vi "send_trigger.vi"(8 "error in (no error)":errorcluster, 11 "GenericStimulator in":refnum<class "GenericStimulator.lvclass">) -> (0 "error out":errorcluster, 3 "GenericStimulator out":refnum<class "GenericStimulator.lvclass">)   [LabVIEW 2010, in "GenericStimulator.lvclass"]
uses:
  GenericStimulator.lvclass
  trigger_enum.ctl
  common/classes/GenericToplevelComponent/GenericToplevelComponent/trigger_type_enum.ctl
panel:
  in  "trigger":T1
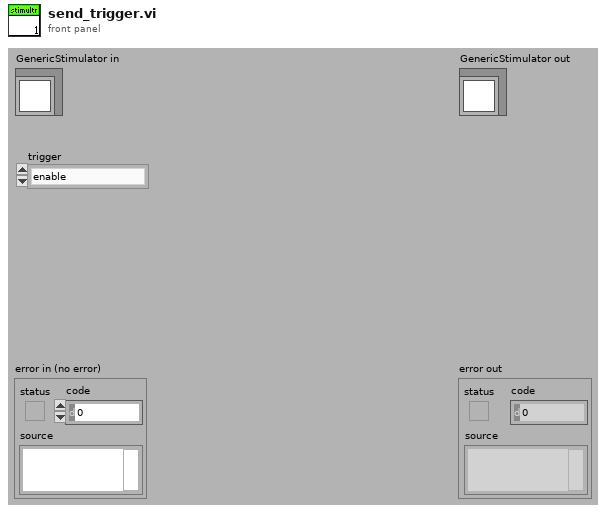
[diagram p1: front panel]
types:
  T1 = typedef "GenericStimulator.lvclass/trigger_enum.ctl" = enum16{"enable", "disable"}
  T2 = typedef "trigger_type_enum.ctl" = enum8{"external", "internal", "common"}
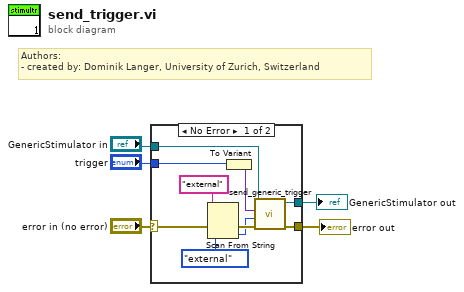
[diagram p0: block diagram]
diagram:
  # "Authors: \n- created by: Dominik Langer, University of Zurich, Switzerland"
  n1 = case shown="No Error" "error in (no error)" {
    selector: "error in (no error)" -> [w9 w17]
    tunnel: [w12 w17] -> w3
    tunnel: [w13 w16] -> w4
    tunnel: "GenericStimulator in" -> [w14 w16]
    tunnel: "trigger" -> [w15 _]
    frame No Error {
      n2 = Scan From String(input string="external", error in=w9, default 1=trigger_type_enum."external" ("trigger type")) -> (error out=w8:errorcluster, output 1=w7:T2)  [unwired: 2 in, 2 out]
      n3 = To Variant(anything=w15) -> (Variant=w11:variant)
      n4 = call-dynamic "send_generic_trigger.vi"("error in (no error)"=w8, "trigger type"=w7, "trigger variant"=w11, "GenericToplevelComponent in"=w14) -> ("error out"=w12:errorcluster, "GenericToplevelComponent out"=w13:refnum<class "GenericStimulator.lvclass">)  [unwired: 4 in, 2 out]
    }
    frame Error {
    }
  }
  "error out" <- w3
  "GenericStimulator out" <- w4
